vi "demo - auto-index ascii for loop.vi"() -> ()   [LabVIEW 2024]
doc: "#vi_description \nGenerate an ASCII table\nThetic Engineering Ltd."
uses:
  <vilib>/Analysis/1siggen.llb/Ramp Pattern by Delta.vi
  <vilib>/Analysis/NI_AALBase.lvlib
panel:
  out "current iteration":i32
  out "ASCII Table":string[][](table)
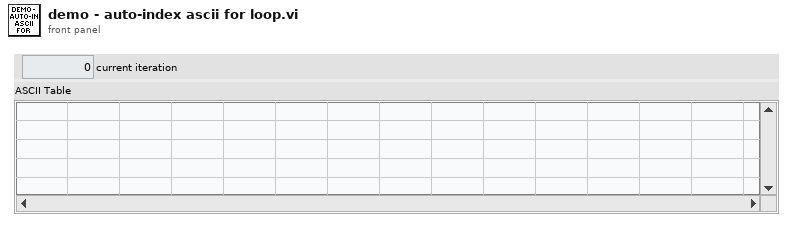
[diagram p1: front panel]
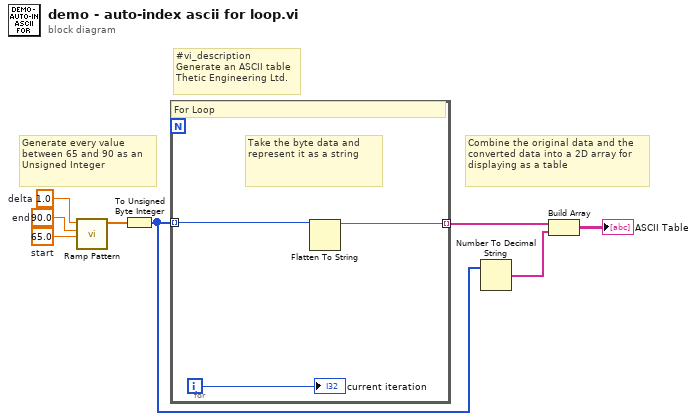
[diagram p0: block diagram]
diagram:
  w6 = 1.0  # delta
  w7 = 90.0  # end
  w8 = 65.0  # start
  # "Combine the original data and the converted data into a 2D array for displaying as a table"
  # "Generate every value between 65 and 90 as an Unsigned Integer"
  # "#vi_description \nGenerate an ASCII table\nThetic Engineering Ltd."
  n1 = call-poly <vilib>:"Ramp Pattern.vi"("start"=w8, "end"=w7, "delta"=w6) -> ("Ramp Pattern"=w5:dbl[])  [unwired: 6 in, 2 out]
  n2 = To Unsigned Byte Integer(number=w5) -> (unsigned 8bit integer=w2:u8[])
  n3 = for {
    tunnel: w2 -> [w10] mode=indexing
    tunnel: [w9] -> w4 mode=indexing
    i -> [w11]
    # "Take the byte data and represent it as a string"
    # "For Loop"
    n4 = Flatten To String(anything=w10) -> (data string=w9:string)  [unwired: 3 in, 2 out]
    "current iteration" <- w11
  }
  n5 = Number To Decimal String(number=w2) -> (decimal integer string=w1:string[])  [unwired: 1 in]
  n6 = Build Array(w4, w1) -> (→"ASCII Table":string[][])
